vi "ex_4_5.vi"() -> ()   [LabVIEW 2020]
panel:
  in  "Word":string
  out "Result text":string
  in  "Original text":string
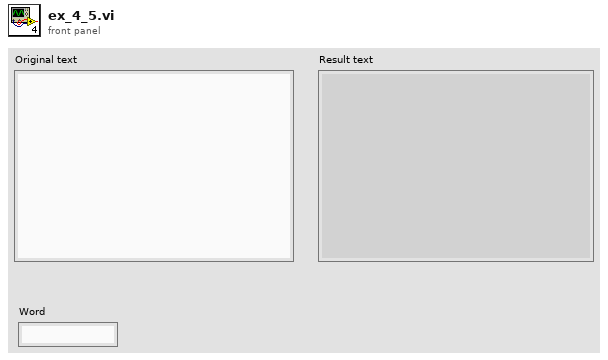
[diagram p1: front panel]
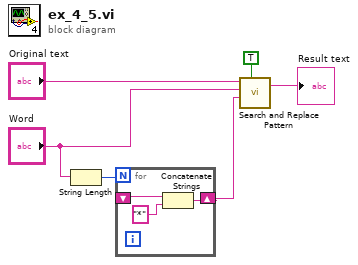
[diagram p0: block diagram]
diagram:
  n1 = String Length(string="Word") -> (length=w3:i32)
  n2 = for {
    N: w3 -> [_]
    shift-right: [w8] -> w2
    shift-left: _ -> [w7]
    n3 = Concatenate Strings(w7, "*" ("replace string (\"\")")) -> (w8:string)
  }
  n4 = call <vilib>:"Search and Replace Pattern.vi"("string"="Original text", "regular expression (\"\")"="Word", "replace string (\"\")"=w2, "replace all? (F)"=TRUE) -> ("result string"=→"Result text":string)  [unwired: 1 in, 1 out]
